vi "camera initialization.vi"(0 "Camera SPIMB":T1={"Horizontal Offset"=1000, "Vertical Offset"=772, "Horizontal Width"=500, "Vertical Width"=500}, 6 "Force Open":bool, 7 "error in (no error)":errorcluster {"code" format="%.0x"}, 14 "Camera SPIMA":T1={"Horizontal Offset"=1000, "Vertical Offset"=772, "Horizontal Width"=500, "Vertical Width"=500}) -> (1 "SPIMB Out":u32, 4 "SPIMB Error":errorcluster={"status"=TRUE, "code"=-2113925119, "source"="TMERR_UNKNOWNERROR - An unknown error has occurred at C:\\Program Files\\National Instruments\\LabVIEW 2015\\user.lib\\Hamamatsu Video Capture\\tm_opencamera.vi"}, 5 "SPIMB Serial No":string, 15 "SPIMA Out":u32=1, 18 "SPIMA Error":errorcluster={"status"=TRUE, "code"=-2113925119, "source"="TMERR_UNKNOWNERROR - An unknown error has occurred at C:\\Program Files\\National Instruments\\LabVIEW 2015\\user.lib\\Hamamatsu Video Capture\\tm_opencamera.vi"}, 19 "SPIMA Serial No":string)   [LabVIEW 2016]
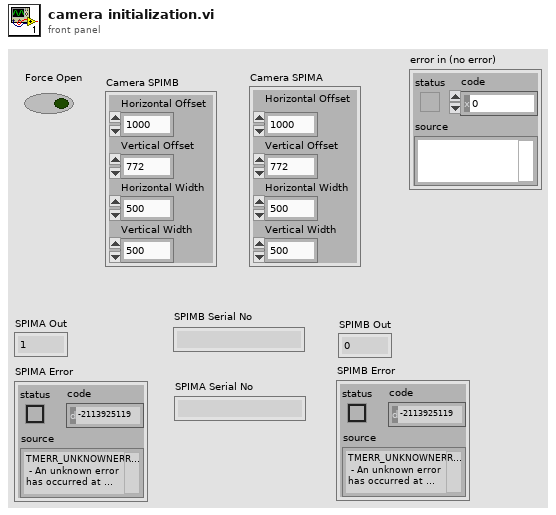
[diagram p1: front panel]
types:
  T1 = cluster{"Horizontal Offset":i32, "Vertical Offset":i32, "Horizontal Width":i32, "Vertical Width":i32}
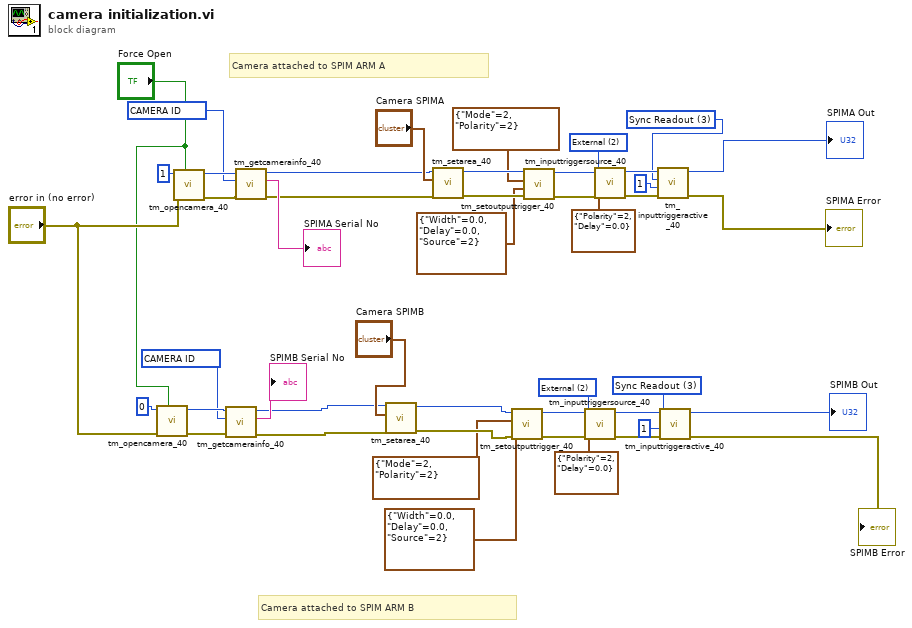
[diagram p0: block diagram]
diagram:
  w2 = 2 items=["Internal"=1, "External"=2, "Software"=3, "Master Pulse"=4] ("Source")
  w4 = 3 items=["Edge"=1, "Level"=2, "Sync Readout"=3, "Point"=4] ("Active")
  w12 = 3 items=["Edge"=1, "Level"=2, "Sync Readout"=3, "Point"=4] ("Active")
  w18 = 2 items=["Internal"=1, "External"=2, "Software"=3, "Master Pulse"=4] ("Source")
  w39 = u32 67109122 items=["BUS"=67109121, "CAMERA ID"=67109122, "VENDOR"=67109123, "MODEL"=67109124, "CAMERA VERSION"=67109125, "DRIVER VERSION"=67109126, "MODULE VERSIOIN"=67109127, "DCAMAPI VERSION"=67109128] ("Info ID")
  w42 = u32 67109122 items=["BUS"=67109121, "CAMERA ID"=67109122, "VENDOR"=67109123, "MODEL"=67109124, "CAMERA VERSION"=67109125, "DRIVER VERSION"=67109126, "MODULE VERSIOIN"=67109127, "DCAMAPI VERSION"=67109128] ("Info ID")
  # "Camera attached to SPIM ARM A"
  # "Camera attached to SPIM ARM B"
  n1 = call <userlib>:"tm_opencamera_40.vi"("Force Open"="Force Open", "error in (no error)"="error in (no error)", "Camera Index"=u32 0) -> ("error out"=w40:errorcluster, "Handle out"=w41:u32)  [unwired: 6 in, 1 out]
  n2 = call <userlib>:"tm_opencamera_40.vi"("Force Open"="Force Open", "error in (no error)"="error in (no error)", "Camera Index"=u32 1) -> ("error out"=w43:errorcluster, "Handle out"=w44:u32)  [unwired: 6 in, 1 out]
  n3 = call <userlib>:"tm_getcamerainfo_40.vi"("error in (no error)"=w40, "Info ID"=w39, "Handle in"=w41) -> ("error out"=w33:errorcluster, "String"=→"SPIMB Serial No":string, "Handle out"=w34:u32)  [unwired: 6 in]
  n4 = call <userlib>:"tm_getcamerainfo_40.vi"("error in (no error)"=w43, "Info ID"=w42, "Handle in"=w44) -> ("error out"=w31:errorcluster, "String"=→"SPIMA Serial No":string, "Handle out"=w32:u32)  [unwired: 6 in]
  n5 = call <userlib>:"tm_setarea_40.vi"("error in (no error)"=w33, "Sub Region"="Camera SPIMB", "Handle in"=w34) -> ("error out"=w26:errorcluster, "Handle out"=w27:u32)  [unwired: 7 in]
  n6 = call <userlib>:"tm_setarea_40.vi"("error in (no error)"=w31, "Sub Region"="Camera SPIMA", "Handle in"=w32) -> ("error out"=w28:errorcluster, "Handle out"=w29:u32)  [unwired: 7 in]
  n7 = call <userlib>:"tm_setoutputtrigger_40.vi"("error in (no error)"=w26, "Programmable Options"=cluster{"Width":dbl, "Delay":dbl, "Source":u32} {"Width"=0.0, "Delay"=0.0, "Source"=2}, "Type"=cluster{"Mode":u32, "Polarity":u32} {"Mode"=2, "Polarity"=2}, "Handle in"=w27) -> ("error out"=w9:errorcluster, "Handle out"=w10:u32)  [unwired: 6 in]
  n8 = call <userlib>:"tm_setoutputtrigger_40.vi"("error in (no error)"=w28, "Programmable Options"=cluster{"Width":dbl, "Delay":dbl, "Source":u32} {"Width"=0.0, "Delay"=0.0, "Source"=2}, "Type"=cluster{"Mode":u32, "Polarity":u32} {"Mode"=2, "Polarity"=2}, "Handle in"=w29) -> ("error out"=w19:errorcluster, "Handle out"=w20:u32)  [unwired: 6 in]
  n9 = call <userlib>:"tm_inputtriggersource_40.vi"("error in (no error)"=w9, "External Options"=cluster{"Polarity":i32, "Delay":dbl} {"Polarity"=2, "Delay"=0.0}, "Source"=w2, "Handle in"=w10) -> ("error out"=w7:errorcluster, "Handle out"=w8:u32)  [unwired: 6 in]
  n10 = call <userlib>:"tm_inputtriggersource_40.vi"("error in (no error)"=w19, "External Options"=cluster{"Polarity":i32, "Delay":dbl} {"Polarity"=2, "Delay"=0.0}, "Source"=w18, "Handle in"=w20) -> ("error out"=w15:errorcluster, "Handle out"=w16:u32)  [unwired: 6 in]
  n11 = call <userlib>:"tm_inputtriggeractive_40.vi"("error in (no error)"=w15, "Times"=1, "Active"=w12, "Handle in"=w16) -> ("error out"=→"SPIMA Error":errorcluster, "Handle out"=→"SPIMA Out":u32)  [unwired: 6 in]
  n12 = call <userlib>:"tm_inputtriggeractive_40.vi"("error in (no error)"=w7, "Times"=1, "Active"=w4, "Handle in"=w8) -> ("error out"=→"SPIMB Error":errorcluster, "Handle out"=→"SPIMB Out":u32)  [unwired: 6 in]
